vi "Radau5_Weighted Norm for Z.vi"(10 "Tolerance Vector":dbl[](array[numeric]), 11 "Increment of Z":dbl[](array[numeric])) -> (3 "Norm of  Z":dbl)   [LabVIEW 2017, in "NI_DAE.lvlib"]
uses:
  <vilib>/gmath/NI_DAE.lvlib
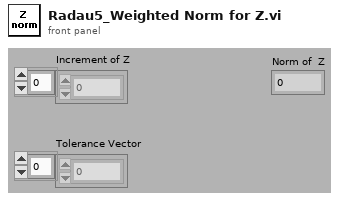
[diagram p1: front panel]
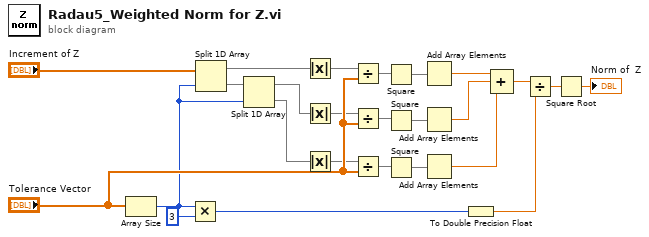
[diagram p0: block diagram]
diagram:
  n1 = Array Size(array="Tolerance Vector") -> (size(s)=w5:i32)
  n2 = Multiply(x=w5, y=3) -> (x*y=w12:i32)
  n3 = Split 1D Array(array="Increment of Z", index=w5) -> (first subarray=w8:dbl[], second subarray=w10:dbl[])
  n4 = Split 1D Array(array=w10, index=w5) -> (first subarray=w7:dbl[], second subarray=w6:dbl[])
  n5 = Absolute Value(x=w8) -> (abs(x)=w22:dbl[])
  n6 = Absolute Value(x=w7) -> (abs(x)=w21:dbl[])
  n7 = Absolute Value(x=w6) -> (abs(x)=w20:dbl[])
  n8 = Divide(x=w22, y="Tolerance Vector") -> (x/y=w23:dbl[])
  n9 = Divide(x=w21, y="Tolerance Vector") -> (x/y=w19:dbl[])
  n10 = Divide(x=w20, y="Tolerance Vector") -> (x/y=w18:dbl[])
  n11 = Square(x=w23) -> (x^2=w16:dbl[])
  n12 = Square(x=w19) -> (x^2=w15:dbl[])
  n13 = Square(x=w18) -> (x^2=w14:dbl[])
  n14 = Add Array Elements(numeric array=w16) -> (sum=w4:dbl)
  n15 = Add Array Elements(numeric array=w15) -> (sum=w3:dbl)
  n16 = Add Array Elements(numeric array=w14) -> (sum=w2:dbl)
  n17 = To Double Precision Float(number=w12) -> (double precision float=w11:dbl)
  n18 = Compound Arithmetic op=ADD(w4, w3, w2) -> (w1:dbl)
  n19 = Divide(x=w1, y=w11) -> (x/y=w17:dbl)
  n20 = Square Root(x=w17) -> (sqrt(x)=→"Norm of  Z":dbl)
